vi "stateAction.vi"(8 "error in (no error)":errorcluster, 11 "Context in":refnum<class "Context.lvclass">) -> (0 "error out":errorcluster, 3 "Context out":refnum<class "Context.lvclass">)   [LabVIEW 2018, in "Context.lvclass"]
uses:
  Context.lvclass
  Context.lvclass/Context.ctl
  State/State.lvclass
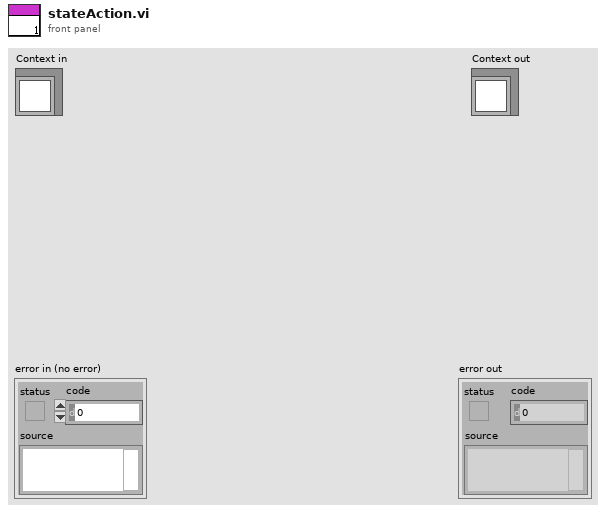
[diagram p1: front panel]
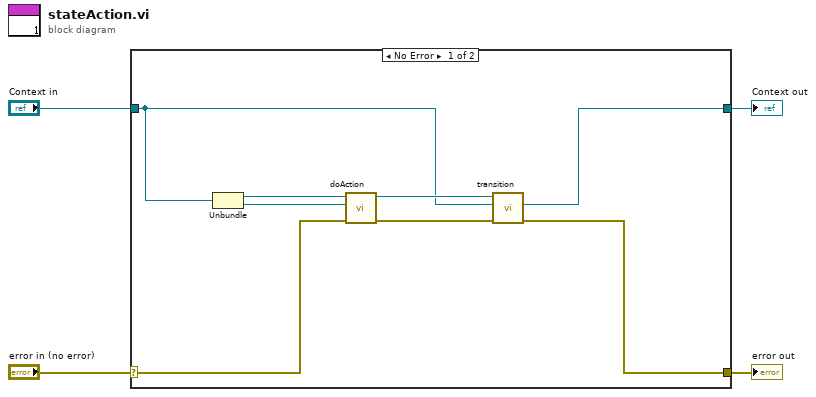
[diagram p0: block diagram]
diagram:
  n1 = case shown="No Error" "error in (no error)" {
    selector: "error in (no error)" -> [w12 w14]
    tunnel: [w9 w14] -> w3
    tunnel: [w6 w13] -> w1
    tunnel: "Context in" -> [w7 w13]
    frame No Error {
      n2 = Unbundle(w7) -> (w10:refnum<class "State.lvclass">, w5:refnum<class "ContextData.lvclass">)
      n3 = call-dynamic "doAction.vi"("error in (no error)"=w12, "ContextData"=w5, "State in"=w10) -> ("error out"=w11:errorcluster, "State out"=w8:refnum<class "State.lvclass">)  [unwired: 7 in]
      n4 = call-dynamic "transition.vi"("error in (no error)"=w11, "Context In"=w7, "State in"=w8) -> ("error out"=w9:errorcluster, "Context Out"=w6:refnum<class "Context.lvclass">)  [unwired: 6 in, 1 out]
    }
    frame Error {
    }
  }
  "error out" <- w3
  "Context out" <- w1
